vi "Read Test Execs.vi"(11 "Parallel in":refnum<class "Parallel.lvclass">) -> (2 "Test Execs":refnum<data-value>[](array[refnum]), 3 "Parallel out":refnum<class "Parallel.lvclass">)   [LabVIEW 2019, in "Test Executive.lvlib" / "Parallel.lvclass"]
uses:
  <vilib>/gpm_packages/@cs/test-executive/Source/Test Executive/Parallel/Parallel.lvclass
  <vilib>/gpm_packages/@cs/test-executive/Source/Test Executive/ITestExecutive/ITest Executive.lvclass
  <vilib>/gpm_packages/@cs/test-executive/Source/Test Executive/Parallel/Parallel.lvclass/Parallel.ctl
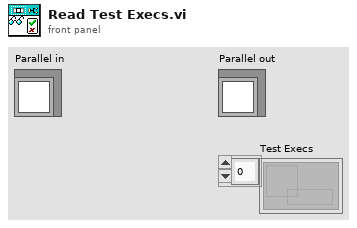
[diagram p1: front panel]
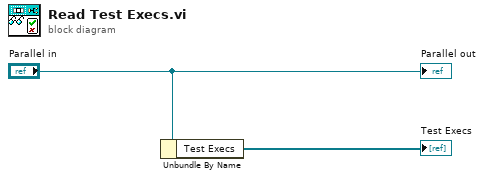
[diagram p0: block diagram]
diagram:
  n1 = Unbundle By Name("Parallel in") -> ("Test Execs"=→"Test Execs":refnum<data-value>[])
  "Parallel out" <- "Parallel in"
